vi "Write Tests.vi"(10 "Tests":T1, 11 "IED Test in":refnum<class "IED Test.lvclass">) -> (3 "IED Test out":refnum<class "IED Test.lvclass">)   [LabVIEW 2018, in "IED Test Framework.lvlib" / "IED Test.lvclass"]
uses:
  IED Test.lvclass
  Controls/Tests Cluster.ctl
  IED Test.lvclass/IED Test.ctl
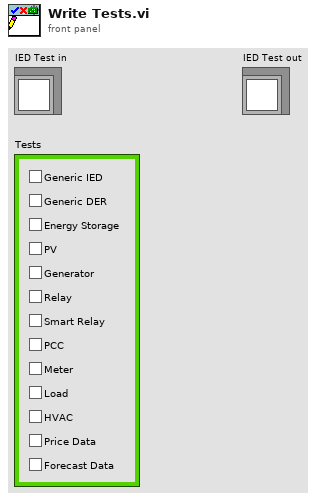
[diagram p1: front panel]
types:
  T1 = typedef "IED Test Framework.lvlib/IED Test.lvclass/Tests Cluster.ctl" = cluster{"Generic IED":bool, "Generic DER":bool, "Energy Storage":bool, "PV":bool, "Generator":bool, "Relay":bool, "Smart Relay":bool, "PCC":bool, "Meter":bool, "Load":bool, "HVAC":bool, "Price Data":bool, "Forecast Data":bool}
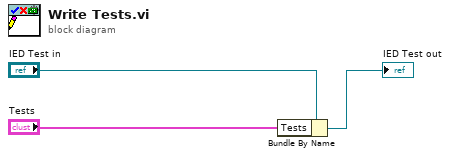
[diagram p0: block diagram]
diagram:
  n1 = Bundle By Name(cluster="IED Test in", "Tests"="Tests") -> (→"IED Test out":refnum<class "IED Test.lvclass">)
